vi "Export files.vi"(8 "Error In":errorcluster, 11 "INI ref in":T1) -> (0 "Error Out":errorcluster, 3 "INI ref out":T1)   [LabVIEW 2015]
uses:
  <vilib>/Utility/config.llb/Config Data RefNum.ctl
  Utilities/Export state.ctl
  <vilib>/Utility/sysdir.llb/System Directory Type.ctl
  <vilib>/Utility/config.llb/Read Key (Path).vi
  <vilib>/Utility/config.llb/NI_LVConfig.lvlib
panel:
  in  "Overwrite?":bool
  out "Success":string caption="Config Message"
  in  "Open":bool
  in  "Cancel":bool
  in  "Export":bool
  in  "Folder path":path
  in  "File types":enum16{"Data Files", "Record Files"}(ring)
  # "Please select the files to export, and select a folder\nto export them to. The folder will be created\nautomatically if it didn't already exist."
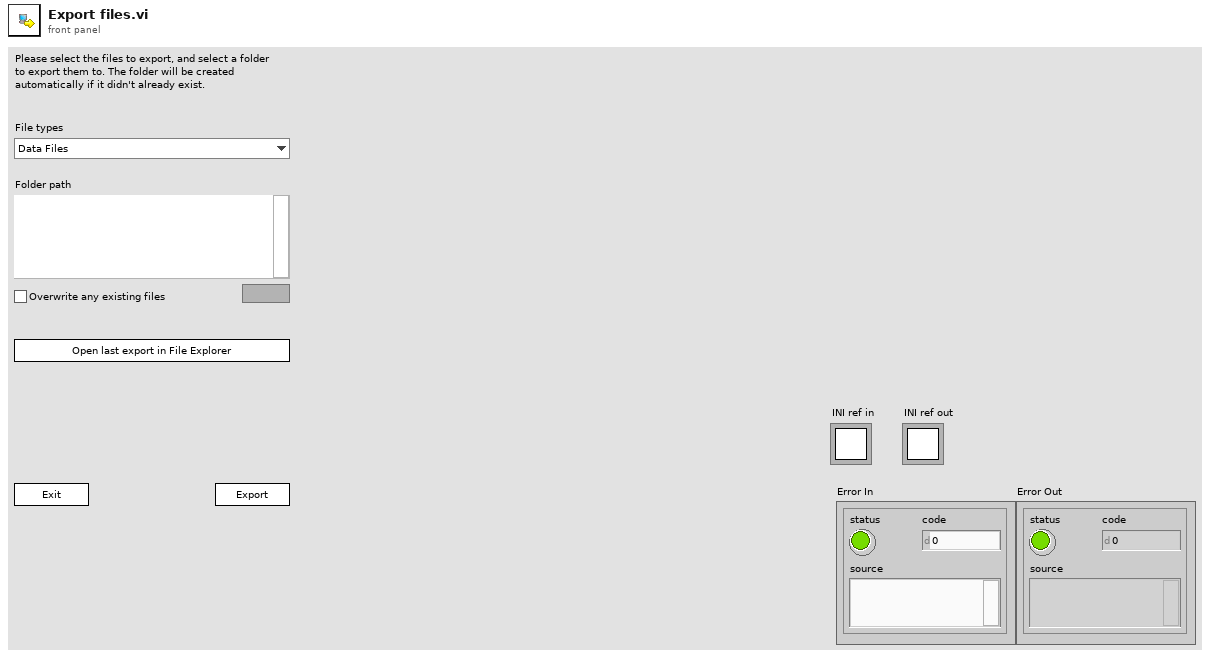
[diagram p1: front panel]
types:
  T1 = typedef "NI_LVConfig.lvlib/Config Data RefNum.ctl" = refnum<k1>
  T2 = typedef "Export state.ctl" = enum16{"Init", "Idle", "Copy data", "Copy records", "Open folder", "Exit"}
  T3 = enum8{"Enabled", "Disabled", "Disabled and Grayed Out"}
  T4 = typedef "System Directory Type.ctl" = i32
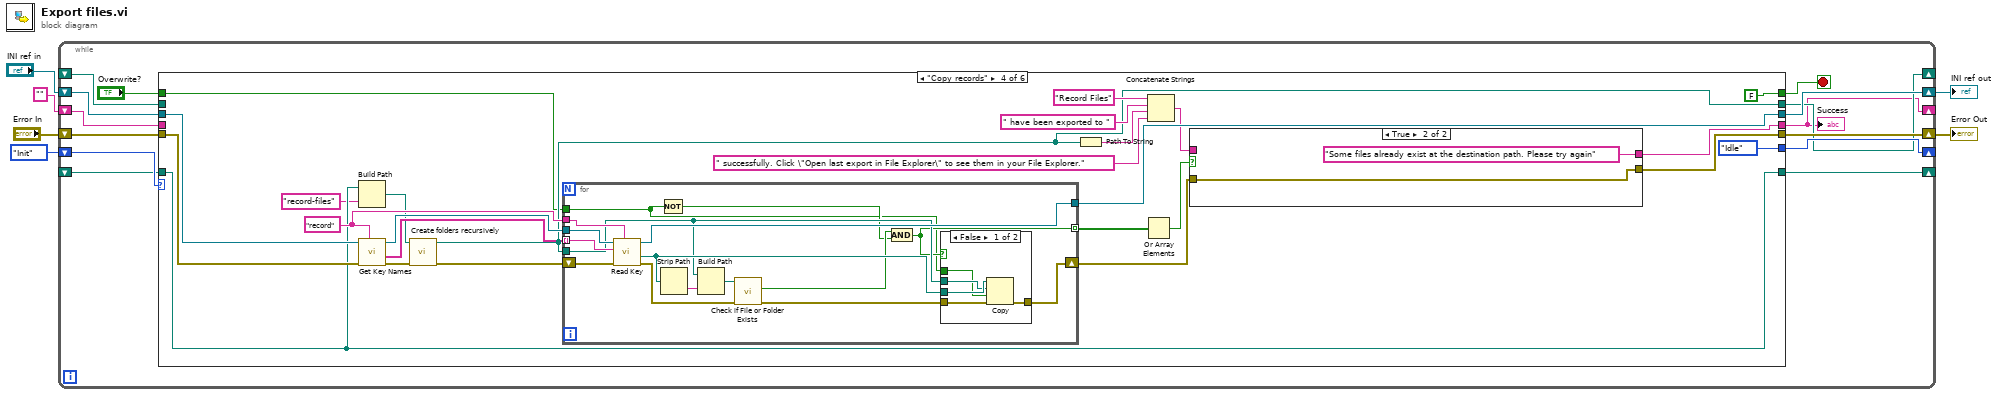
[diagram p0: block diagram]
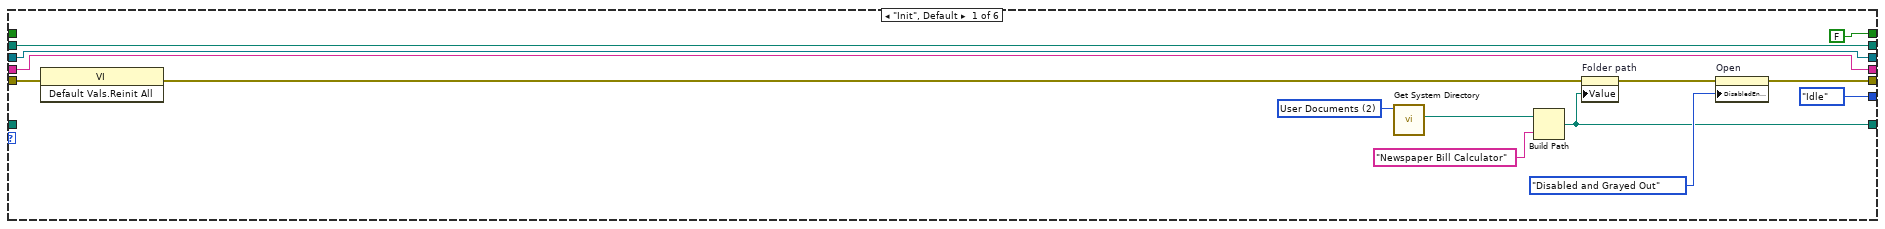
[diagram p2: hidden frame]
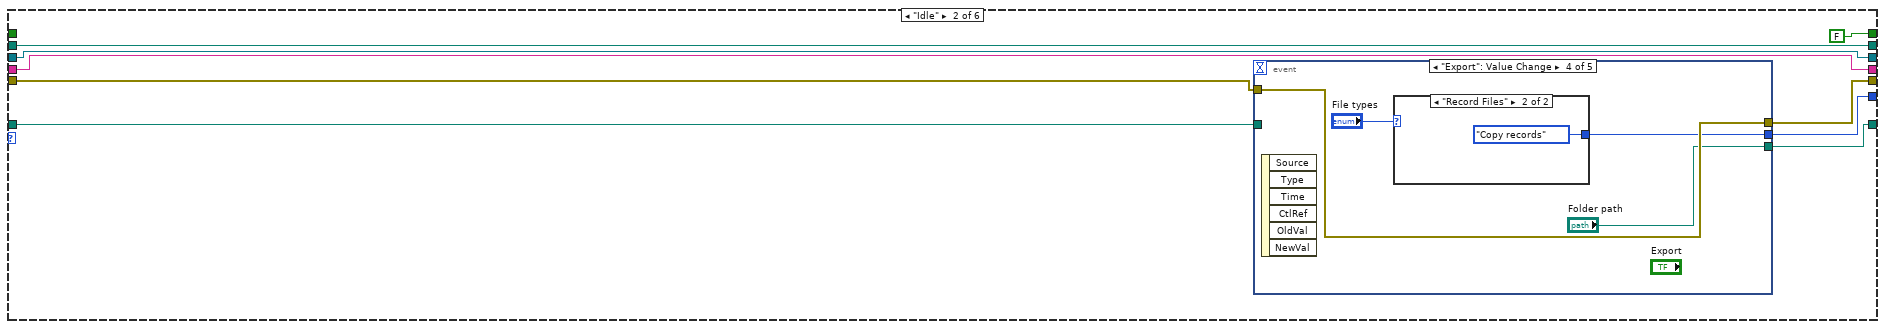
[diagram p3: hidden frame]
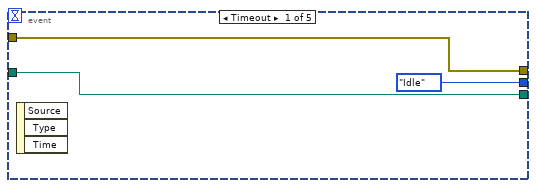
[diagram p4: hidden frame]
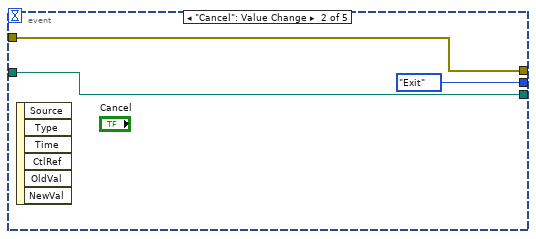
[diagram p5: hidden frame]
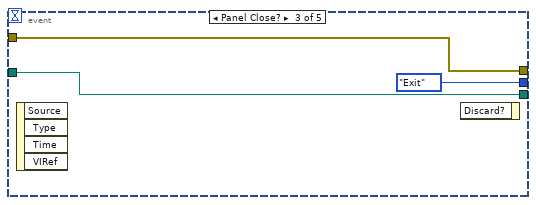
[diagram p6: hidden frame]
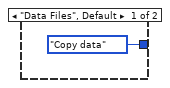
[diagram p7: hidden frame]
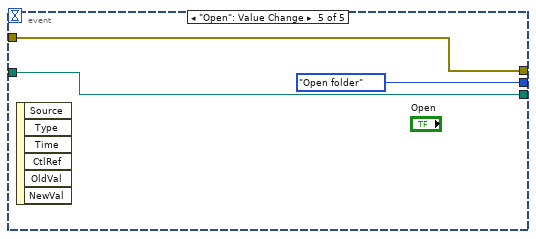
[diagram p8: hidden frame]
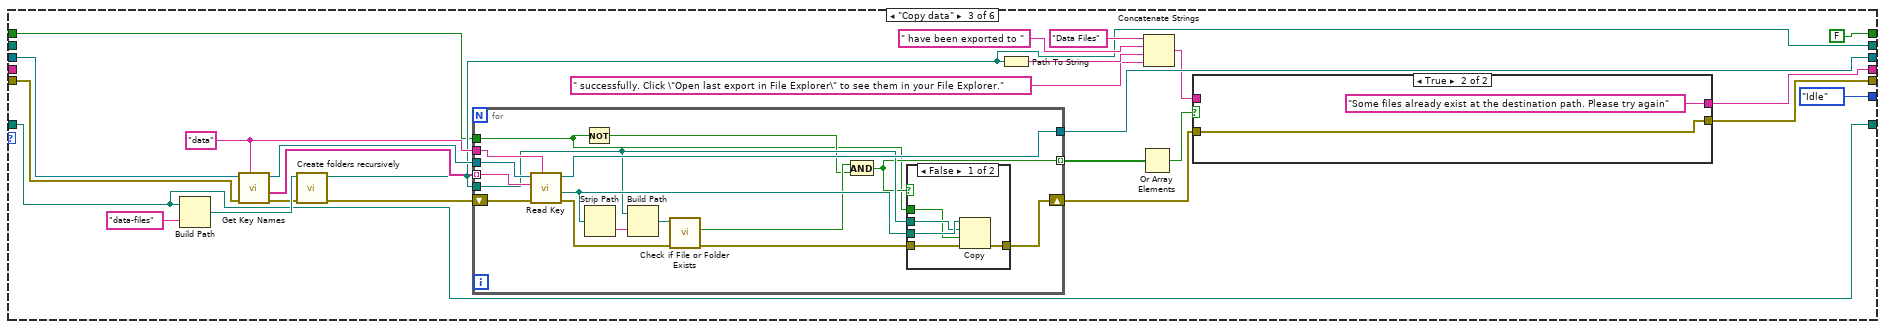
[diagram p9: hidden frame]
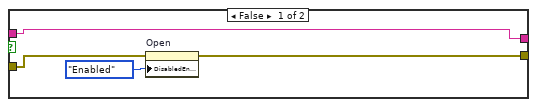
[diagram p10: hidden frame]
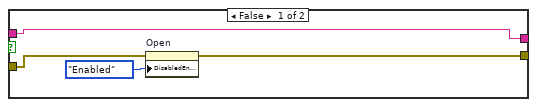
[diagram p12: hidden frame]
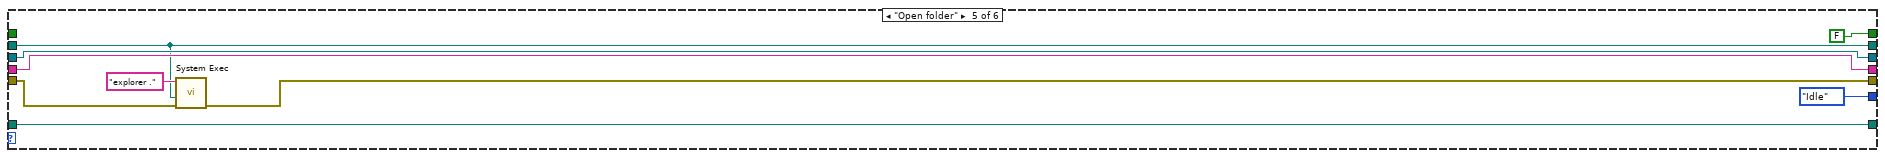
[diagram p14: hidden frame]
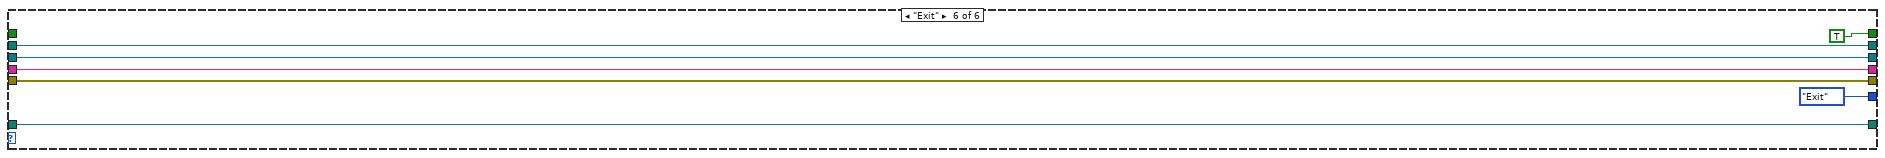
[diagram p15: hidden frame]
diagram:
  n1 = while {
    shift-right: [w19] -> _
    shift-left: Export_state."Init" -> [w20]
    shift-right: [w17] -> w4
    shift-left: "Error In" -> [w18]
    shift-right: [w15] -> _
    shift-left: _ -> [w14]
    shift-right: [w13] -> w2
    shift-left: "INI ref in" -> [w16]
    shift-right: [w12] -> _
    shift-left: _ -> [w11]
    shift-right: [w10] -> _
    shift-left: "" -> [w9]
    stop <- w8 stop-if-true
    n2 = case shown="\"Copy records\"" w20 {
      tunnel: [Export_state."Idle" w43 Export_state."Idle" Export_state."Idle" Export_state."Idle" Export_state."Exit"] -> w19
      tunnel: w18 -> [w30 w41 w85 w138 w175 w181]
      tunnel: [w28 w42 w65 w118 w170 w181] -> w17
      tunnel: [FALSE FALSE FALSE FALSE FALSE TRUE] -> w8
      tunnel: w16 -> [w23 w36 w86 w139 w173 w182]
      tunnel: [w25 w40 w80 w133 w174 w180] -> w15
      tunnel: w14 -> [_ w39 w80 w133 w174 w180]
      tunnel: [w23 w36 w77 w130 w173 w182] -> w13
      tunnel: [w24 w38 w70 w123 w168 w179] -> w12
      tunnel: w11 -> [w24 w38 _ _ w168 w179]
      tunnel: [w22 w35 w69 w122 w169 w178] -> w10
      tunnel: w9 -> [w22 w35 _ _ w169 w178]
      tunnel: "Overwrite?" -> [_ _ w62 w115 _ _]
      frame "Init", Default {
        w33 = T4 2 items=["User Home"=0, "User Desktop"=1, "User Documents"=2, "User Application Data"=3, "User Preferences"=4, "User Temporary"=5, "Public Documents"=6, "Public Application Data"=7, "Public Preferences"=8, "Public Cache"=13, "System Core Libraries"=9, "System Installed Libraries"=10, "Application Files"=11, "Boot Volume Root"=12] ("system directory type")
        n3 = invoke class="VI" method="Default Vals.Reinit All"(error in=w30) -> (error out=w21:errorcluster)  [unwired: 2 in, 2 out]
        n4 = call <vilib>:"Get System Directory.vi"("system directory type"=w33) -> ("system directory"=w32:path)  [unwired: 10 in]
        n5 = Build Path(base path=w32, name or relative path="Newspaper Bill Calculator") -> (appended path=w25:path)
        n6 = property on="Folder path" class="Path"(error in=w21, "Value"=w25) -> (error out=w29:errorcluster)  [unwired: 1 in, 1 out]
        n7 = property on="Open" class="Bool"(error in=w29, "DisabledEnum"=T3."Disabled and Grayed Out" ("Disabled")) -> (error out=w28:errorcluster)  [unwired: 1 in, 1 out]
      }
      frame "Idle" {
        n8 = event shown="[3] \"Export\": Value Change" {
          selector: _ -> [_ _ _ _ _]
          dyn-events: _ -> [_ _ _ _ _]
          timeout: _ -> [_ _ _ _ _]
          tunnel: [Export_state."Idle" Export_state."Exit" Export_state."Exit" w54 Export_state."Open folder"] -> w43
          tunnel: [w45 w48 w51 w56 w60] -> w42
          tunnel: w41 -> [w45 w48 w51 w56 w60]
          tunnel: [w44 w47 w50 "Folder path" w59] -> w40
          tunnel: w39 -> [w44 w47 w50 _ w59]
          event Timeout {
            n9 = event-data() -> ()  [unwired: 1 in, 3 out]
          }
          event "Cancel": Value Change {
            n10 = event-data() -> ()  [unwired: 1 in, 6 out]
          }
          event Panel Close? {
            n11 = event-data() -> ()  [unwired: 1 in, 4 out]
            n12 = event-data() -> ()  [unwired: 2 in, 1 out]
          }
          event "Export": Value Change {
            n13 = event-data() -> ()  [unwired: 1 in, 6 out]
            n14 = case shown="\"Record Files\"" "File types" {
              tunnel: [Export_state."Copy data" Export_state."Copy records"] -> w54
              frame "Data Files", Default {
              }
              frame "Record Files" {
              }
            }
          }
          event "Open": Value Change {
            n15 = event-data() -> ()  [unwired: 1 in, 6 out]
          }
        }
      }
      frame "Copy data" {
        w82 = "data" ("section")
        n16 = Build Path(base path=w80, name or relative path="data-files" ("section")) -> (appended path=w81:path)
        n17 = call <vilib>:"Get Key Names.vi"("section"=w82, "error in (no error)"=w85, "refnum"=w86) -> ("error out"=w76:errorcluster, "key names"=w83:string[], "refnum out"=w84:T1)  [unwired: 5 in, 1 out]
        n18 = call "Create folders recursively.vi"("error in (no error)"=w76, "Path in"=w81) -> ("error out"=w75:errorcluster, "Path out"=w70:path)  [unwired: 8 in]
        n19 = for {
          tunnel: w84 -> [w108]
          tunnel: w83 -> [w107] mode=indexing
          tunnel: w82 -> [w105]
          shift-right: [w102] -> w66
          shift-left: w75 -> [w106]
          tunnel: [w101] -> w77
          tunnel: w70 -> [w100]
          tunnel: [w96] -> w64 mode=indexing
          tunnel: w62 -> [w93]
          n20 = call-poly <vilib>:"Read Key.vi"("section"=w105, "error in (no error)"=w106, "key"=w107, "refnum"=w108) -> ("error out"=w104:errorcluster, "value"=w103:path, "refnum out"=w101:T1)  [unwired: 4 in, 1 out]
          n21 = Not(x=w93) -> (.not. x?=w94:bool)
          n22 = Strip Path(path=w103) -> (name=w97:string)  [unwired: 1 out]
          n23 = Build Path(base path=w100, name or relative path=w97) -> (appended path=w98:path)
          n24 = call <vilib>:"Check if File or Folder Exists.vi"("error in (no error)"=w104, "path"=w98) -> ("error out"=w99:errorcluster, "file or folder exists?"=w95:bool)  [unwired: 7 in, 1 out]
          n25 = And(x=w95, y=w94) -> (x .and. y?=w96:bool)
          n26 = case shown="False" w96 {
            tunnel: w103 -> [w113 _]
            tunnel: [w112 w114] -> w102
            tunnel: w100 -> [w111 _]
            tunnel: w99 -> [w110 w114]
            tunnel: w93 -> [w109 _]
            frame False {
              n27 = Copy(8:w110, 9:w109, 10:w111, 11:w113) -> (0:w112:errorcluster)  [unwired: 1 in, 2 out]
            }
            frame True {
            }
          }
        }
        n28 = Path To String(path=w70) -> (string=w72:string)
        n29 = Or Array Elements(Boolean array=w64) -> (logical OR=w67:bool)
        n30 = Concatenate Strings("Data Files" ("name or relative path"), " have been exported to " ("string"), w72, " successfully. Click \"Open last export in File Explorer\" to see them in your File Explorer." ("string")) -> (w68:string)
        n31 = case shown="True" w67 {
          tunnel: [w90 "Some files already exist at the destination path. Please try again"] -> w69
          tunnel: w68 -> [w90 _]
          tunnel: w66 -> [w89 w91]
          tunnel: [w88 w91] -> w65
          frame False {
            n32 = property on="Open" class="Bool"(error in=w89, "DisabledEnum"=T3."Enabled" ("Disabled")) -> (error out=w88:errorcluster)  [unwired: 1 in, 1 out]
          }
          frame True {
          }
        }
      }
      frame "Copy records" {
        w135 = "record" ("section")
        n33 = Build Path(base path=w133, name or relative path="record-files" ("section")) -> (appended path=w134:path)
        n34 = call <vilib>:"Get Key Names.vi"("section"=w135, "error in (no error)"=w138, "refnum"=w139) -> ("error out"=w129:errorcluster, "key names"=w136:string[], "refnum out"=w137:T1)  [unwired: 5 in, 1 out]
        n35 = call "Create folders recursively.vi"("error in (no error)"=w129, "Path in"=w134) -> ("error out"=w128:errorcluster, "Path out"=w123:path)  [unwired: 8 in]
        n36 = for {
          tunnel: w137 -> [w161]
          tunnel: w136 -> [w160] mode=indexing
          tunnel: w135 -> [w158]
          shift-right: [w155] -> w119
          shift-left: w128 -> [w159]
          tunnel: [w154] -> w130
          tunnel: w123 -> [w153]
          tunnel: [w149] -> w117 mode=indexing
          tunnel: w115 -> [w146]
          n37 = call-poly <vilib>:"Read Key.vi"("section"=w158, "error in (no error)"=w159, "key"=w160, "refnum"=w161) -> ("error out"=w157:errorcluster, "value"=w156:path, "refnum out"=w154:T1)  [unwired: 4 in, 1 out]
          n38 = Not(x=w146) -> (.not. x?=w147:bool)
          n39 = Strip Path(path=w156) -> (name=w150:string)  [unwired: 1 out]
          n40 = Build Path(base path=w153, name or relative path=w150) -> (appended path=w151:path)
          n41 = call <vilib>:"Check if File or Folder Exists.vi"("error in (no error)"=w157, "path"=w151) -> ("error out"=w152:errorcluster, "file or folder exists?"=w148:bool)  [unwired: 7 in, 1 out]
          n42 = And(x=w148, y=w147) -> (x .and. y?=w149:bool)
          n43 = case shown="False" w149 {
            tunnel: w156 -> [w166 _]
            tunnel: [w165 w167] -> w155
            tunnel: w153 -> [w164 _]
            tunnel: w152 -> [w163 w167]
            tunnel: w146 -> [w162 _]
            frame False {
              n44 = Copy(8:w163, 9:w162, 10:w164, 11:w166) -> (0:w165:errorcluster)  [unwired: 1 in, 2 out]
            }
            frame True {
            }
          }
        }
        n45 = Path To String(path=w123) -> (string=w125:string)
        n46 = Or Array Elements(Boolean array=w117) -> (logical OR=w120:bool)
        n47 = Concatenate Strings("Record Files" ("name or relative path"), " have been exported to " ("string"), w125, " successfully. Click \"Open last export in File Explorer\" to see them in your File Explorer." ("string")) -> (w121:string)
        n48 = case shown="True" w120 {
          tunnel: [w143 "Some files already exist at the destination path. Please try again"] -> w122
          tunnel: w121 -> [w143 _]
          tunnel: w119 -> [w142 w144]
          tunnel: [w141 w144] -> w118
          frame False {
            n49 = property on="Open" class="Bool"(error in=w142, "DisabledEnum"=T3."Enabled" ("Disabled")) -> (error out=w141:errorcluster)  [unwired: 1 in, 1 out]
          }
          frame True {
          }
        }
      }
      frame "Open folder" {
        n50 = call <vilib>:"System Exec.vi"("error in (no error)"=w175, "working directory"=w168, "command line"="explorer .") -> ("error out"=w170:errorcluster)  [unwired: 5 in, 3 out]
      }
      frame "Exit" {
      }
    }
    "Success" <- w10
  }
  "INI ref out" <- w2
  "Error Out" <- w4
